vi "MotorEncoder_Loop.vi"(2 "Error In":errorcluster, 3 "MotorEncoderTasks":refnum<k21>[](array[refnum])) -> (0 "Error Out":errorcluster, 1 "MotorEncoderTasks dup":refnum<k21>[](array[refnum]))   [LabVIEW 2015]
uses:
  <vilib>/Platform/TimedLoop/XDataNode/timing_clust.ctl
  <vilib>/Platform/TimedLoop/XDataNode/nitl_modes.ctl
  <vilib>/Platform/TimedLoop/XDataNode/wakeup.ctl
  <vilib>/DAQmx/read.llb/DAQmx Read (Counter DBL 1Chan 1Samp).vi
  <vilib>/DAQmx/miscellaneous.llb/DAQmx Fill In Error Info.vi
  <vilib>/Platform/TimedLoop/XDataNode/XDataNode.xnode
  <vilib>/Platform/TimedLoop/XDataNode/XDNodeRunTimeDep.lvlib
  Shared Libraries/CustomVIs/CustomVI.lvlib
panel:
  out "MotorCableLength(m)":dbl[](array[numeric])
  in  "TransferRatio(m/rev)":dbl=0.22
  out "EncAngles(deg)":dbl[](array[numeric])
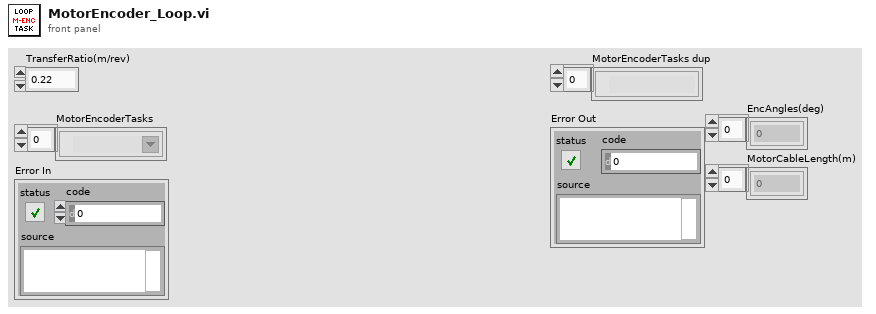
[diagram p1: front panel]
types:
  T1 = typedef "XDNodeRunTimeDep.lvlib/timing_clust.ctl" = cluster{"Expected End [f-1]":u64, "Actual End [f-1]":u64, "Finished Late? [f-1]":bool, "Expected End [i-1]":u64, "Actual End [i-1]":u64, "Finished Late? [i-1]":bool, "Expected Start [i]":u64, "Actual Start [i]":u64, "Expected Start [f]":u64, "Actual Start [f]":u64, "Source Name":string, "Structure Name":string, "Period":i64, "Deadline":i64, "Offset":i64, "Start":i64, "Priority":i32, "Timeout":i32, "Mode":T2, "Wakeup Reason":T3, "Error":errorcluster, "Source Type":string, "Secondary Source Type":string, "Global End Time":u64, "Global Start Time":u64, "Frame Duration":u64, "Iteration Duration":u64, "Assigned CPU":i32, "I/O Scan Engine Mode":u32}
  T2 = typedef "XDNodeRunTimeDep.lvlib/nitl_modes.ctl" = enum32{"No Change", "Process missed periods, maintain original phase", "Discard missed periods, maintain original phase", "Process missed periods, ignore original phase", "Discard missed periods, ignore original phase"}
  T3 = typedef "XDNodeRunTimeDep.lvlib/wakeup.ctl" = enum32{"Normal", "Aborted", "Asynchronous wakeup", "Timing source error", "Timed loop error", "Timeout"}
  T4 = cluster{"Input":enum16{"Fr:Cable", "Fr:Motor", "Fr:Sensor"}, "Output":enum16{"To:Cable", "To:Motor", "To:Sensor"}}
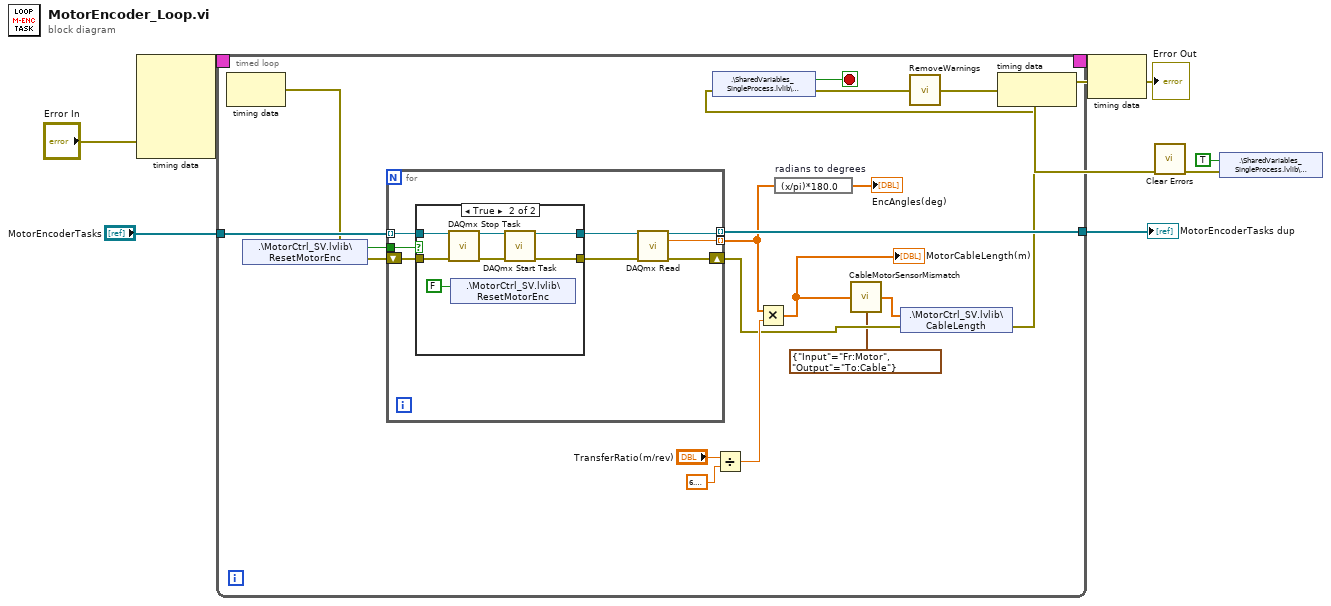
[diagram p0: block diagram]
diagram:
  n1 = node-c288("Error In") -> (w8:T1)  [unwired: 4 in]
  n2 = timed-loop {
    timing: w8 -> [_]
    timing-out: [_] -> w7
    tunnel: "MotorEncoderTasks" -> [w26]
    tunnel: [w23] -> w4
    stop <- w17 stop-if-true
    n3 = node-c288() -> (w24:errorcluster)  [unwired: 1 in]
    n4 = shared-variable ".\\MotorCtrl_SV.lvlib\\ResetMotorEnc"(error in=w24) -> (w25:bool, error out=w16:errorcluster)
    n5 = for {
      tunnel: w26 -> [w34] mode=indexing
      tunnel: w25 -> [w33]
      tunnel: [w30] -> w22 mode=indexing
      tunnel: [w29] -> w23 mode=indexing
      shift-right: [w28] -> w15
      shift-left: w16 -> [w27]
      n6 = case shown="True" w33 {
        tunnel: w34 -> [w36 w43]
        tunnel: w27 -> [w35 w41]
        tunnel: [w35 w39] -> w31
        tunnel: [w36 w38] -> w32
        frame False {
        }
        frame True {
          n7 = call <vilib>:"DAQmx Stop Task.vi"("task/channels in"=w43, "error in"=w41) -> ("task out"=w42:refnum<k21>, "error out"=w40:errorcluster)  [unwired: 12 in]
          n8 = shared-variable ".\\MotorCtrl_SV.lvlib\\ResetMotorEnc"(FALSE) -> ()  [unwired: 1 in, 1 out]
          n9 = call <vilib>:"DAQmx Start Task.vi"("task/channels in"=w42, "error in"=w40) -> ("task out"=w38:refnum<k21>, "error out"=w39:errorcluster)  [unwired: 12 in]
        }
      }
      n10 = call-poly <vilib>:"DAQmx Read.vi"("task/channels in"=w32, "error in"=w31) -> ("task out"=w29:refnum<k21>, "data"=w30:dbl, "error out"=w28:errorcluster)  [unwired: 11 in]
    }
    n11 = Divide(x="TransferRatio(m/rev)", y=6.283185307179586) -> (x/y=w18:dbl)
    n12 = Multiply(x=w22, y=w18) -> (x*y=w13:dbl[])
    "MotorCableLength(m)" <- w13
    n13 = expression code="(x/pi)*180.0" "radians to degrees"(w22) -> (→"EncAngles(deg)":dbl[])
    n14 = call "CableMotorSensorMismatch.vi"("Conversion"=T4 {"Input"=enum."Fr:Motor", "Output"=enum."To:Cable"}, "Input"=w13) -> ("Output"=w12:dbl[])  [unwired: 2 in]
    n15 = shared-variable ".\\MotorCtrl_SV.lvlib\\CableLength"(w12, error in=w15) -> (error out=w14:errorcluster)
    n16 = shared-variable ".\\SharedVariables_SingleProcess.lvlib\\GlobalStop"(error in=w14) -> (w17:bool, error out=w10:errorcluster)
    n17 = call "RemoveWarnings.vi"("error in (no error)"=w10) -> ("error out"=w9:errorcluster)
    n18 = node-c288(w9) -> ()  [unwired: 1 out]
  }
  "MotorEncoderTasks dup" <- w4
  n19 = node-c288(w7) -> (w2:errorcluster)
  "Error Out" <- w2
  n20 = call <vilib>:"Clear Errors.vi"("error in (no error)"=w2) -> ("error out"=w1:errorcluster)  [unwired: 5 in, 1 out]
  n21 = shared-variable ".\\SharedVariables_SingleProcess.lvlib\\GlobalStop"(TRUE ("GlobalStop"), error in=w1) -> ()  [unwired: 1 out]
